vi "Update Other Clients.vi"(10 "data string":string, 11 "TCP Network Connection in":refnum<k5>) -> ()   [LabVIEW 2017]
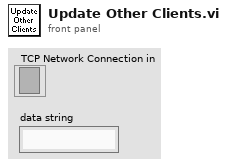
[diagram p1: front panel]
types:
  T1 = enum16{"Add Cnx", "Remove Cnx", "Retrieve List", "Cnx Inited"}
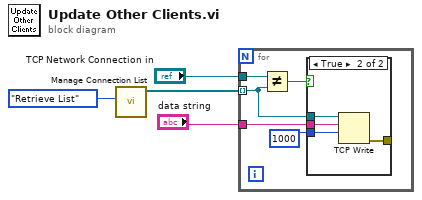
[diagram p0: block diagram]
diagram:
  n1 = call <vilib>:"Manage Connection List.vi"("Operation"=T1."Retrieve List") -> ("Connections List"=w2:refnum<k5>[])  [unwired: 8 in, 2 out]
  n2 = for {
    tunnel: "TCP Network Connection in" -> [w9]
    tunnel: "data string" -> [w8]
    tunnel: w2 -> [w6] mode=indexing
    n3 = Not Equal?(x=w9, y=w6) -> (x != y?=w7:bool)
    n4 = case shown="True" w7 {
      tunnel: w8 -> [_ w13]
      tunnel: w6 -> [_ w12]
      tunnel: 1000 -> [_ w11]
      tunnel: [_ w10] -> _
      frame False {
      }
      frame True {
        n5 = TCP Write(connection ID=w12, data in=w13, 9:w11) -> (error out=w10:errorcluster)  [unwired: 1 in, 2 out]
      }
    }
  }
